vi "KepcoDCPwr Initialize.vi"(0 "VISA Resource Name":refnum<visa-resource-name>, 2 "recognize device (True)":bool=TRUE caption="Recognize Device (True)", 5 "Model":string, 7 "id query (True)":bool=TRUE, 9 "reset device (True)":bool=TRUE, 11 "error in (no error)":errorcluster {"code" format="%.0x"}) -> (4 "VISA Session Out":refnum<visa-resource-name>, 6 "Model Out":string, 13 "Raw Model":string, 15 "error out":errorcluster {"code" format="%.0x"})   [LabVIEW 2020]
doc: "This VI performs the following initialization actions:\n\n- Creates a new VISA session.\n\n- Opens a session to the specified device using the interface and address you specify for the Resource Name parameter.\n\n- If the ID Query parameter is set to TRUE, this VI queries the instrument ID and checks that it is valid for this instrument driver.\n\n- If the Reset parameter is set to TRUE, this VI resets the instrument to a known state.\n\n- Sends initialization commands to set the instrument to the state necessary for the operation of the instrument driver.\n\n- Returns an instrument handle that you use to identify the instrument in all subsequent instrument driver VI calls.\n\nNote: This VI creates a new session each time you invoke it. Although you can open more than one VISA session for the same resource, it is best not to do so. You can use the same session in multiple program threads."
uses:
  Match Regular Expression.xnode
panel:
  out "idn length":u32
  out "Interface Information:Interface Type":u16(ring)=1 items=["GPIB"=1, "VXI"=2, "GPIB-VXI"=3, "Serial"=4, "PXI"=5, "TCPIP"=6, "USB"=7, "FireWire"=9]
  out "Interface Type":string
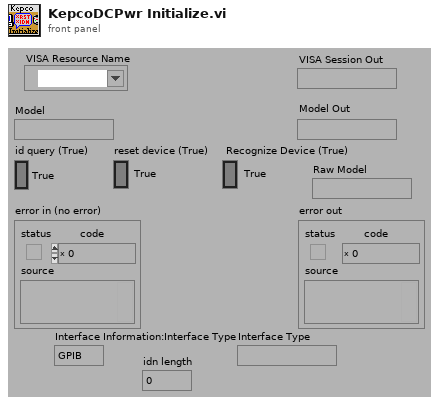
[diagram p1: front panel]
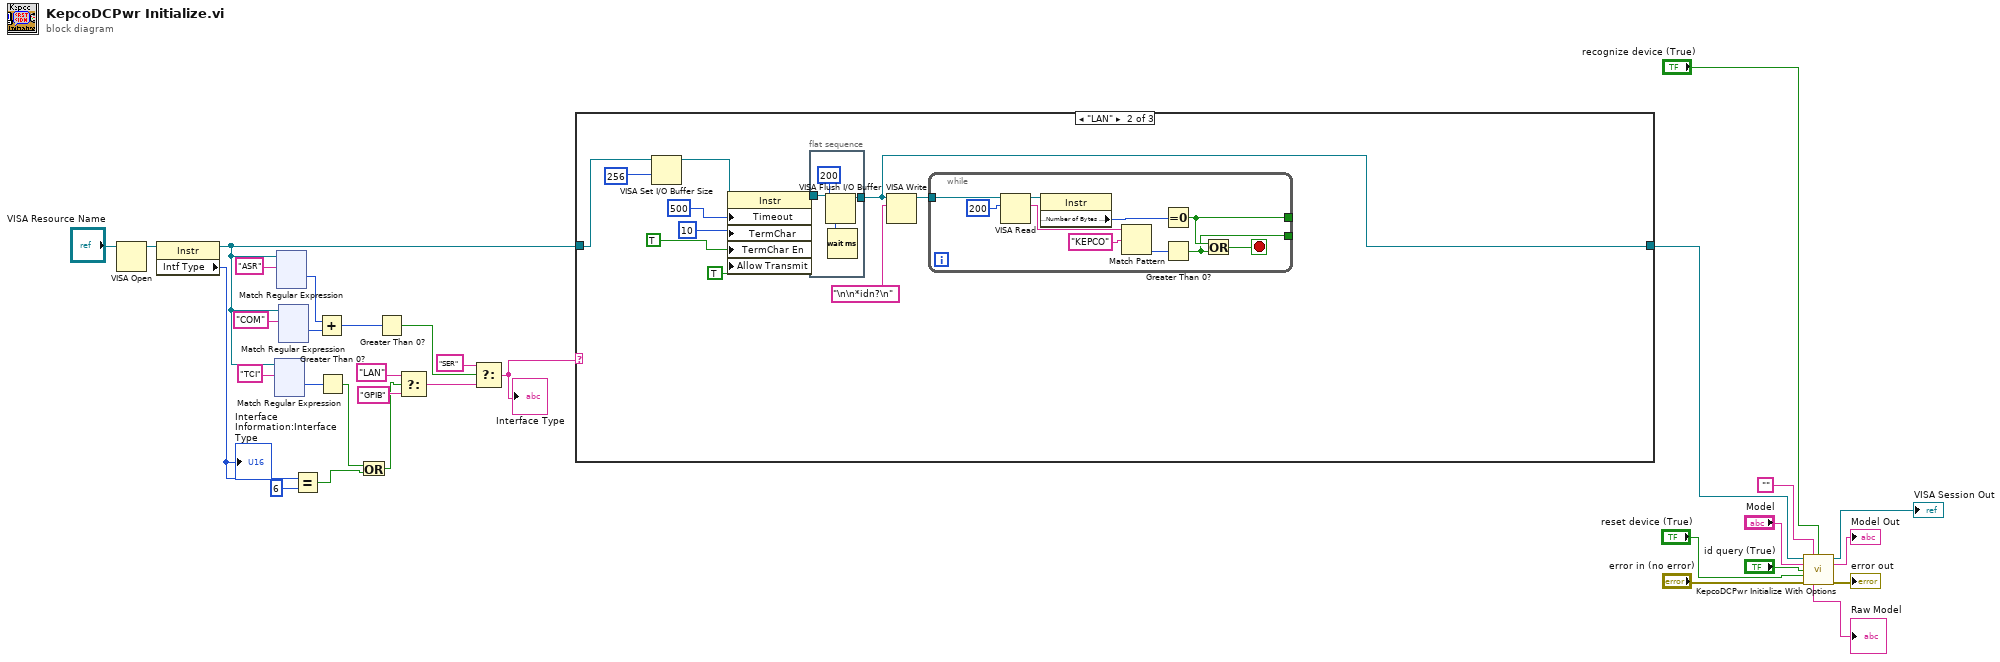
[diagram p0: block diagram]
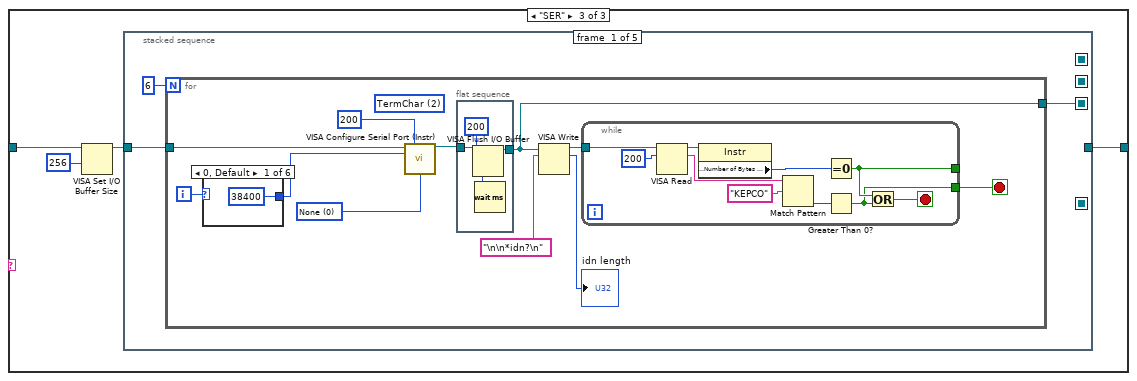
[diagram p3: hidden frame]
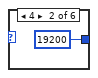
[diagram p4: hidden frame]
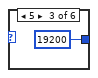
[diagram p5: hidden frame]
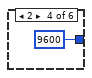
[diagram p6: hidden frame]
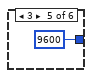
[diagram p7: hidden frame]
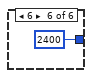
[diagram p8: hidden frame]
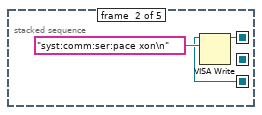
[diagram p9: hidden frame]
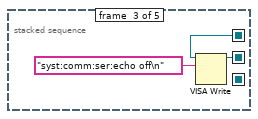
[diagram p10: hidden frame]
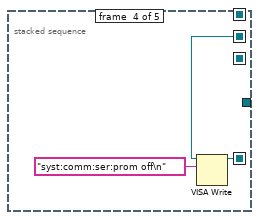
[diagram p11: hidden frame]
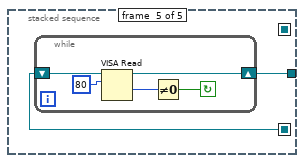
[diagram p12: hidden frame]
diagram:
  n1 = VISA Open(VISA resource name="VISA Resource Name") -> (VISA resource name=w7:refnum<visa-resource-name>)  [unwired: 4 in, 1 out]
  n2 = property class="Instr"(reference=w7) -> (reference out=w6:refnum<visa-resource-name>, "Intf Type"=w5:u16)  [unwired: 1 in, 1 out]
  "Interface Information:Interface Type" <- w5
  n3 = xnode "Match Regular Expression"("input string"=w6, "regular expression"="TCI") -> ("offset past match"=w13:i32)  [unwired: 2 in, 6 out]
  n4 = xnode "Match Regular Expression"("input string"=w6, "regular expression"="ASR") -> ("offset past match"=w19:i32)  [unwired: 2 in, 6 out]
  n5 = xnode "Match Regular Expression"("input string"=w6, "regular expression"="COM") -> ("offset past match"=w16:i32)  [unwired: 2 in, 6 out]
  n6 = Equal?(x=w5, y=u16 6) -> (x = y?=w3:bool)
  n7 = Add(x=w19, y=w16) -> (x+y=w18:i32)
  n8 = Greater Than 0?(x=w13) -> (x > 0?=w2:bool)
  n9 = Or(x=w2, y=w3) -> (x .or. y?=w1:bool)
  n10 = Greater Than 0?(x=w18) -> (x > 0?=w17:bool)
  n11 = Select(t="LAN", s=w1, f="GPIB") -> (s? t:f=w12:string)
  n12 = Select(t="SER", s=w17, f=w12) -> (s? t:f=w9:string)
  "Interface Type" <- w9
  n13 = case shown="\"LAN\"" w9 {
    tunnel: [w33 w35 w61] -> w24
    tunnel: w6 -> [w33 w37 w60]
    frame "GPIB", Default {
    }
    frame "LAN" {
      n14 = VISA Set I/O Buffer Size(VISA resource name=w37, size (4096)=u32 256) -> (VISA resource name out=w36:refnum<visa-resource-name>)  [unwired: 2 in, 1 out]
      n15 = property class="Instr"(reference=w36, "Timeout"=500, "TermChar"=10, "TermChar En"=TRUE ("Message Based Settings:Termination Character Enable"), "Allow Transmit"=TRUE ("Serial Settings:Allow Transmit")) -> (reference out=w41:refnum<visa-resource-name>)  [unwired: 1 in, 1 out]
      n16 = flat-sequence {
        tunnel: w41 -> [w47]
        tunnel: [w46] -> w35
        frame #0 {
          n17 = VISA Flush I/O Buffer(VISA resource name=w47) -> (VISA resource name out=w46:refnum<visa-resource-name>)  [unwired: 2 in, 1 out]
          n18 = Wait (ms)(milliseconds to wait=u32 200) -> ()  [unwired: 1 out]
        }
      }
      n19 = VISA Write(VISA resource name=w35, write buffer="\n\n*idn?\n") -> (VISA resource name out=w40:refnum<visa-resource-name>)  [unwired: 1 in, 2 out]
      n20 = while {
        tunnel: w40 -> [w57]
        tunnel: [w50] -> _
        tunnel: [w49] -> _
        stop <- w48 stop-if-true
        n21 = VISA Read(VISA resource name=w57, byte count=u32 200) -> (VISA resource name out=w53:refnum<visa-resource-name>, read buffer=w55:string)  [unwired: 1 in, 2 out]
        n22 = property class="Instr"(reference=w53) -> ("Serial Settings:Number of Bytes at Serial Port"=w52:u32)  [unwired: 1 in, 2 out]
        n23 = Match Pattern(string=w55, regular expression="KEPCO") -> (offset past match=w51:i32)  [unwired: 1 in, 3 out]
        n24 = Equal To 0?(x=w52) -> (x = 0?=w50:bool)
        n25 = Greater Than 0?(x=w51) -> (x > 0?=w49:bool)
        n26 = Or(x=w50, y=w49) -> (x .or. y?=w48:bool)
      }
    }
    frame "SER" {
      n27 = VISA Set I/O Buffer Size(VISA resource name=w60, size (4096)=u32 256) -> (VISA resource name out=w59:refnum<visa-resource-name>)  [unwired: 2 in, 1 out]
      n28 = stacked-sequence {
        seq-local: [w63 _ _ _ _] -> [_ w96 _ _ _]
        seq-local: [_ w95 _ _ _] -> [_ _ w99 _ _]
        seq-local: [_ _ w98 _ _] -> [_ _ _ w102 _]
        seq-local: [_ _ _ w101 _] -> [_ _ _ _ w105]
        tunnel: w59 -> [w62 _ _ _ _]
        tunnel: [_ _ _ _ w104] -> w61
        frame #0 {
          n29 = for {
            N: 6 -> [_]
            tunnel: w62 -> [w69]
            tunnel: [w73] -> w63
            i -> [w75]
            stop <- w71 stop-if-true
            (unwired) u16 2 items=["None", "Last Bit", "TermChar"] ("Serial Settings:End Mode for Reads")
            w65 = u16 0 items=["None", "XON/XOFF", "RTS/CTS", "XON/XOFF & RTS/CTS", "DTR/DSR", "XON/XOFF & DTR/DSR"] ("Serial Settings:Flow Control")
            n30 = case shown="0, Default" w75 {
              tunnel: [u32 38400 ("Serial Settings:Baud Rate") u32 19200 ("Serial Settings:Baud Rate") u32 19200 ("Serial Settings:Baud Rate") u32 9600 ("Serial Settings:Baud Rate") u32 9600 ("Serial Settings:Baud Rate") u32 2400 ("Serial Settings:Baud Rate")] -> w66
              frame 0, Default {
              }
              frame 4 {
              }
              frame 5 {
              }
              frame 2 {
              }
              frame 3 {
              }
              frame 6 {
              }
            }
            n31 = call "VISA Configure Serial Port (Instr).vi"("VISA resource name"=w69, "timeout (10sec)"=200, "baud rate (9600)"=w66, "flow control (0:none)"=w65) -> ("VISA resource name out"=w68:refnum<visa-resource-name>)  [unwired: 10 in, 1 out]
            n32 = flat-sequence {
              tunnel: w68 -> [w78]
              tunnel: [w77] -> w73
              frame #0 {
                n33 = VISA Flush I/O Buffer(VISA resource name=w78) -> (VISA resource name out=w77:refnum<visa-resource-name>)  [unwired: 2 in, 1 out]
                n34 = Wait (ms)(milliseconds to wait=u32 200) -> ()  [unwired: 1 out]
              }
            }
            n35 = VISA Write(VISA resource name=w73, write buffer="\n\n*idn?\n") -> (VISA resource name out=w74:refnum<visa-resource-name>, return count=→"idn length":u32)  [unwired: 1 in, 1 out]
            n36 = while {
              tunnel: w74 -> [w88]
              tunnel: [w81] -> _
              tunnel: [w80] -> w71
              stop <- w79 stop-if-true
              n37 = VISA Read(VISA resource name=w88, byte count=u32 200) -> (VISA resource name out=w84:refnum<visa-resource-name>, read buffer=w86:string)  [unwired: 1 in, 2 out]
              n38 = property class="Instr"(reference=w84) -> ("Serial Settings:Number of Bytes at Serial Port"=w83:u32)  [unwired: 1 in, 2 out]
              n39 = Match Pattern(string=w86, regular expression="KEPCO") -> (offset past match=w82:i32)  [unwired: 1 in, 3 out]
              n40 = Equal To 0?(x=w83) -> (x = 0?=w81:bool)
              n41 = Greater Than 0?(x=w82) -> (x > 0?=w80:bool)
              n42 = Or(x=w81, y=w80) -> (x .or. y?=w79:bool)
            }
          }
        }
        frame #1 {
          n43 = VISA Write(VISA resource name=w96, write buffer="syst:comm:ser:pace xon\n" ("write buffer (\"\")")) -> (VISA resource name out=w95:refnum<visa-resource-name>)  [unwired: 1 in, 2 out]
        }
        frame #2 {
          n44 = VISA Write(VISA resource name=w99, write buffer="syst:comm:ser:echo off\n" ("write buffer (\"\")")) -> (VISA resource name out=w98:refnum<visa-resource-name>)  [unwired: 1 in, 2 out]
        }
        frame #3 {
          n45 = VISA Write(VISA resource name=w102, write buffer="syst:comm:ser:prom off\n" ("write buffer (\"\")")) -> (VISA resource name out=w101:refnum<visa-resource-name>)  [unwired: 1 in, 2 out]
        }
        frame #4 {
          n46 = while {
            shift-right: [w108] -> w104
            shift-left: w105 -> [w109]
            stop <- w107 continue-if-true
            n47 = VISA Read(VISA resource name=w109, byte count=80) -> (VISA resource name out=w108:refnum<visa-resource-name>, return count=w106:u32)  [unwired: 1 in, 2 out]
            n48 = Not Equal To 0?(x=w106) -> (x != 0?=w107:bool)
          }
        }
      }
    }
  }
  n49 = call "KepcoDCPwr Initialize With Options.vi"("VISA resource name"=w24, "option string (\"Simulate=0,RangeCheck=1,QueryInstrStatus=1,Cache=1\")"="", "recognize device (True)"="recognize device (True)", "Model"="Model", "id query (True)"="id query (True)", "reset device (True)"="reset device (True)", "error in (no error)"="error in (no error)") -> ("VISA Session Out"=→"VISA Session Out":refnum<visa-resource-name>, "Model Out"=→"Model Out":string, "Raw Model"=→"Raw Model":string, "error out"=→"error out":errorcluster)  [unwired: 5 out]
